vi "Create Component Loader.vi"(8 "error in (no error)":errorcluster, 10 "components directory (default)":path, 11 "Component Loader type":refnum<class "Component Loader.lvclass">) -> (0 "error out":errorcluster, 3 "Component Loader out":refnum<class "Component Loader.lvclass">)   [LabVIEW 2017, in "DSF Core.lvlib" / "Component Loader.lvclass"]
uses:
  Component Loader.lvclass
  Component Loader.lvclass/Component Loader.ctl
  VIs/Constants/Default Components Directory.vi
  Component Directory Not Found.vi
  DSF Core.lvlib
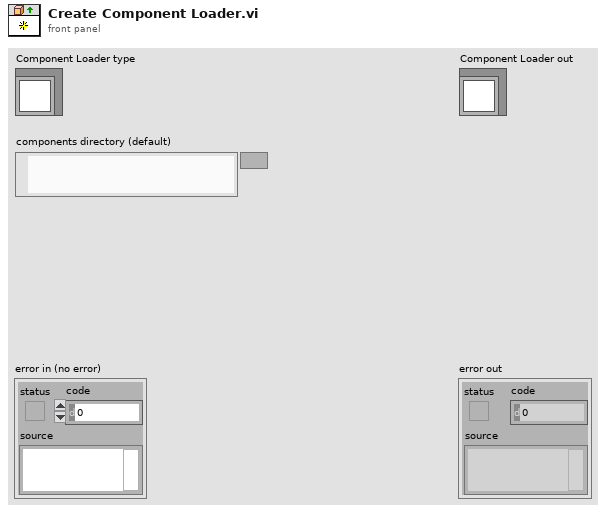
[diagram p1: front panel]
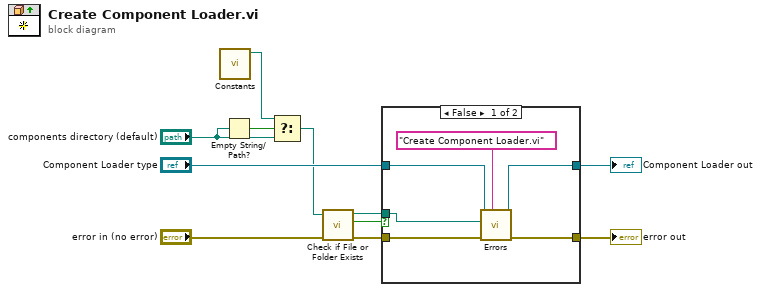
[diagram p0: block diagram]
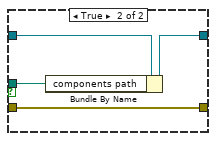
[diagram p2: hidden frame]
diagram:
  n1 = call-poly "Constants.vi"() -> ("Default Components Directory"=w3:path)  [unwired: 11 in]
  n2 = Empty String/Path?(string/path="components directory (default)") -> (empty?=w4:bool)
  n3 = Select(t=w3, s=w4, f="components directory (default)") -> (s? t:f=w1:path)
  n4 = call <vilib>:"Check if File or Folder Exists.vi"("error in (no error)"="error in (no error)", "path"=w1) -> ("error out"=w7:errorcluster, "file or folder exists?"=w5:bool, "dup path"=w8:path)  [unwired: 7 in]
  n5 = case shown="False" w5 {
    tunnel: "Component Loader type" -> [w15 w21]
    tunnel: [w14 w20] -> w10
    tunnel: w8 -> [w13 w19]
    tunnel: w7 -> [w17 w18]
    tunnel: [w16 w18] -> w6
    frame False {
      n6 = call-poly "Errors.vi"("error source vi name"="Create Component Loader.vi", "error in (no error)"=w17, "configured path"=w13, "Component Loader in"=w15) -> ("error out"=w16:errorcluster, "Component Loader out"=w14:refnum<class "Component Loader.lvclass">)  [unwired: 6 in]
    }
    frame True {
      n7 = Bundle By Name(cluster=w21, "components path"=w19) -> (w20:refnum<class "Component Loader.lvclass">)
    }
  }
  "error out" <- w6
  "Component Loader out" <- w10
